vi "use to update setpoints datastructure.vi"() -> ()   [LabVIEW 2015]
uses:
  setpoints.ctl
  backwash.ctl
  coag.ctl
  model type.ctl
  ini.ctl
  file paths.ctl
  <vilib>/Utility/config.llb/NI_LVConfig.lvlib
panel:
  in  "ini":T1=enum."read"
  out "Setpoints out":T2={"graph data interval (s)"=100.0, "sludge flow [L/s]"=0.0, "plant flow [L/s]"=0.0, "Plant Flow PID "={"proportional gain (Kc)"=0.05, "integral time (Ti, min)"=1.0, "derivative time (Td, min)"=0.01}, "Sludge PID "={"proportional gain (Kc)"=0.07, "integral time (Ti, min)"=1.0, "derivative time (Td, min)"=0.01}, "backwash"={"Filtered quality target [NTU]"=0.3, "min filtration time [s]"=600.0, "Ripen time [s]"=600.0}, "Coagulant"={"flocculator volume (L)"=0.0, "clarifier volume (L)"=0.0, "dose updates per HRT"=100, "target clarified turbidity (NTU)"=0.3, "Coagulant mode"=enum."manual", "Coag dose [mg/L]"=0.0, "pump mL/rev"=0.0, "clarifier flow [L/s]"=0.5, "min Coag dose [mg/L]"=0.0, "max Coag dose [mg/L]"=0.0, "Steps"=3, "HRT per ramp update"=1}} {"Coagulant"."HRT per ramp update" min=1 max=10 step=1; "Coagulant"."Steps" min=3 step=1; "Coagulant"."clarifier flow [L/s]" min=0.0001 max=1.0 step=0.0001; "Coagulant"."target clarified turbidity (NTU)" min=0.1 max=5.0 step=0.01; "Coagulant"."dose updates per HRT" min=1 max=100 step=1; "Sludge PID"."derivative time (Td, min)" format="%.3f"; "Sludge PID"."integral time (Ti, min)" format="%.3f"; "Sludge PID"."proportional gain (Kc)" format="%.3f"; "Plant Flow PID"."derivative time (Td, min)" format="%.3f"; "Plant Flow PID"."integral time (Ti, min)" format="%.3f"; "Plant Flow PID"."proportional gain (Kc)" format="%.3f"; "plant flow [L/s]" min=0.05 max=1.0 step=0.05; "sludge flow [L/s]" min=0.0 max=0.05 step=0.001; "graph data interval (s)" min=1 max=1000 step=1}
  out "error out":errorcluster
  in  "setpoints":T2={"graph data interval (s)"=5.0, "sludge flow [L/s]"=0.001, "plant flow [L/s]"=0.5, "Plant Flow PID "={"proportional gain (Kc)"=10.0, "integral time (Ti, min)"=0.4, "derivative time (Td, min)"=0.0}, "Sludge PID "={"proportional gain (Kc)"=0.07, "integral time (Ti, min)"=1.0, "derivative time (Td, min)"=0.01}, "backwash"={"Filtered quality target [NTU]"=0.2, "min filtration time [s]"=3600.0, "Ripen time [s]"=600.0}, "Coagulant"={"flocculator volume (L)"=66.81, "clarifier volume (L)"=2.0, "dose updates per HRT"=10, "target clarified turbidity (NTU)"=0.6, "Coagulant mode"=enum."manual", "Coag dose [mg/L]"=5.5, "pump mL/rev"=0.255, "clarifier flow [L/s]"=0.0033, "min Coag dose [mg/L]"=2.0, "max Coag dose [mg/L]"=6.0, "Steps"=3, "HRT per ramp update"=2}} {"Coagulant"."HRT per ramp update" min=1 max=10 step=1; "Coagulant"."Steps" min=3 step=1; "Coagulant"."clarifier flow [L/s]" min=0.0001 max=1.0 step=0.0001; "Coagulant"."target clarified turbidity (NTU)" min=0.1 max=5.0 step=0.01; "Coagulant"."dose updates per HRT" min=1 max=100 step=1; "Sludge PID"."derivative time (Td, min)" format="%.3f"; "Sludge PID"."integral time (Ti, min)" format="%.3f"; "Sludge PID"."proportional gain (Kc)" format="%.3f"; "Plant Flow PID"."derivative time (Td, min)" format="%.3f"; "Plant Flow PID"."integral time (Ti, min)" format="%.3f"; "Plant Flow PID"."proportional gain (Kc)" format="%.3f"; "plant flow [L/s]" min=0.05 max=1.0 step=0.05; "sludge flow [L/s]" min=0.0 max=0.05 step=0.001; "graph data interval (s)" min=1 max=1000 step=1}
  # "min"
  # "max"
  # "min"
  # "max"
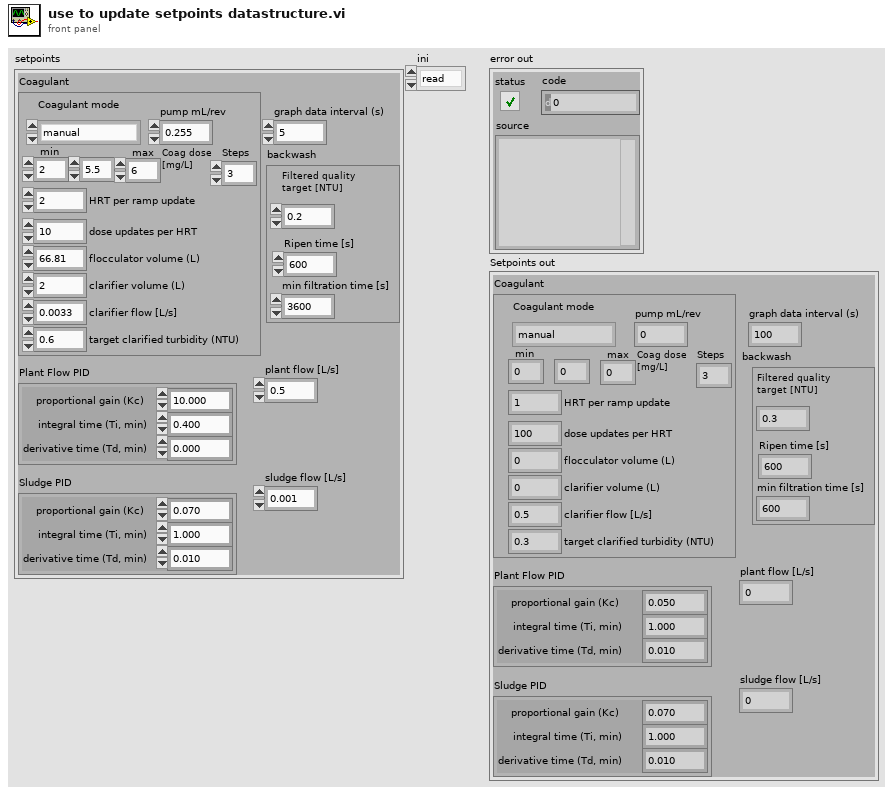
[diagram p1: front panel]
types:
  T1 = typedef "ini.ctl" = enum16{"write", "read"}
  T2 = typedef "setpoints.ctl" = cluster{"graph data interval (s)":sgl, "sludge flow [L/s]":dbl, "plant flow [L/s]":dbl, "Plant Flow PID ":cluster{"proportional gain (Kc)":dbl, "integral time (Ti, min)":dbl, "derivative time (Td, min)":dbl}, "Sludge PID ":cluster{"proportional gain (Kc)":dbl, "integral time (Ti, min)":dbl, "derivative time (Td, min)":dbl}, "backwash":T3, "Coagulant":T4}
  T3 = typedef "backwash.ctl" = cluster{"Filtered quality target [NTU]":dbl, "min filtration time [s]":dbl, "Ripen time [s]":dbl}
  T4 = typedef "coag.ctl" = cluster{"flocculator volume (L)":dbl, "clarifier volume (L)":dbl, "dose updates per HRT":u16, "target clarified turbidity (NTU)":dbl, "Coagulant mode":T5, "Coag dose [mg/L]":dbl, "pump mL/rev":dbl, "clarifier flow [L/s]":dbl, "min Coag dose [mg/L]":dbl, "max Coag dose [mg/L]":dbl, "Steps":u16, "HRT per ramp update":u32}
  T5 = typedef "model type.ctl" = enum16{"manual", "ramp", "simple corrector", "linear regression"}
  T6 = typedef "file paths.ctl" = enum16{"read paths", "close"}
  T7 = typedef "NI_LVConfig.lvlib/Config Data RefNum.ctl" = refnum<k1>
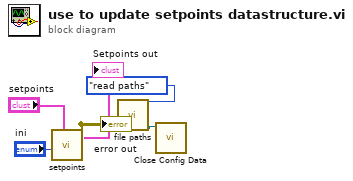
[diagram p0: block diagram]
diagram:
  n1 = call "setpoints.vi"("setpoints"="setpoints", "ini"="ini") -> ("error out"=w2:errorcluster, "Setpoints out"=→"Setpoints out":T2)  [unwired: 8 in]
  "error out" <- w2
  n2 = call "file paths.vi"("error in (no error)"=w2, "file path control"=file_paths."read paths") -> ("ini"=w4:T7)  [unwired: 6 in, 3 out]
  n3 = call <vilib>:"Close Config Data.vi"("refnum"=w4) -> ()  [unwired: 9 in, 2 out]
